vi "Read Serial Settings.vi"(8 "error in":errorcluster, 11 "4124 in":refnum<class "4124.lvclass">) -> (0 "error out":errorcluster, 2 "Serial Configuration":T1={"Baud Rate"=9600, "Parity"=0, "Data Bits"=7, "Stop Bits"=10, "Flow Control"=0} {"Flow Control" items=["None", "XON/XOFF", "RTS/CTS", "XON/XOFF & RTS/CTS", "DTR/DSR", "XON/XOFF & DTR/DSR"]; "Stop Bits" items=["1.0"=10, "1.5"=15, "2.0"=20]; "Data Bits" items=["7"=7, "8"=8]; "Parity" items=["None", "Odd", "Even", "Mark", "Space"]; "Baud Rate" items=["300"=300, "600"=600, "1200"=1200, "2400"=2400, "4800"=4800, "9600"=9600, "19200"=19200]}, 3 "4124 out":refnum<class "4124.lvclass">)   [LabVIEW 2018, in "4124.lvlib" / "4124.lvclass"]
uses:
  4124.lvclass
  builds/Power_Supply.lvlibp/Power Supply.lvclass
  builds/Configuration.lvlibp/Configuration.lvclass
  C:/Users/Ron.Dexter.LUMINARTECH/Desktop/builds/Power_Supply.lvlibp/Power Supply.lvclass
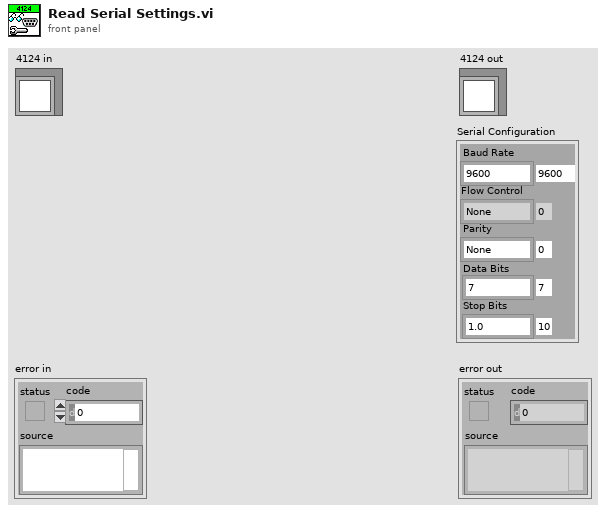
[diagram p1: front panel]
types:
  T1 = cluster{"Baud Rate":u32, "Parity":u16, "Data Bits":u16, "Stop Bits":u16, "Flow Control":u16}
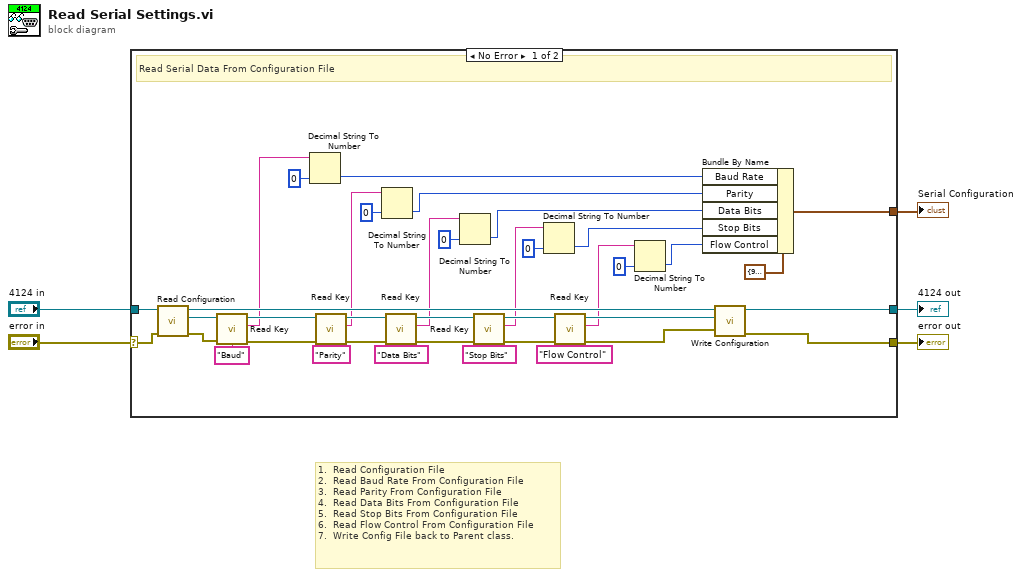
[diagram p0: block diagram]
diagram:
  # "1.  Read Configuration File\n2.  Read Baud Rate From Configuration File\n3.  Read Parity From Configuration File\n4.  Read Data Bits From Configuration File\n5.  Read Stop Bits From Configuration File\n6.  Read Flow Control From Configuration File\n7.  Write Config File back to Parent class."
  n1 = case shown="No Error" "error in" {
    selector: "error in" -> [w20 w46]
    tunnel: [w6 w46] -> w4
    tunnel: [w23 w45] -> w2
    tunnel: "4124 in" -> [w24 w45]
    tunnel: [w21 _] -> w1
    frame No Error {
      # "Read Serial Data From Configuration File"
      n2 = call "Read Configuration.vi"("error in (no error)"=w20, "Power Supply in"=w24) -> ("error out"=w43:errorcluster, "Configuration"=w44:refnum<class "Configuration.lvclass">, "Power Supply out"=w31:refnum<class "4124.lvclass">)  [unwired: 7 in]
      n3 = call "Read Key.vi"("Key:"="Baud", "error in"=w43, "Configuration in"=w44) -> ("error out"=w29:errorcluster, "Value"=w19:string, "Configuration out"=w35:refnum<class "Configuration.lvclass">)  [unwired: 6 in]
      n4 = Decimal String To Number(string=w19, default (0L)=u32 0 ("default (0 I32)")) -> (number=w18:u32)  [unwired: 1 in, 1 out]
      n5 = call "Read Key.vi"("Key:"="Parity", "error in"=w29, "Configuration in"=w35) -> ("error out"=w28:errorcluster, "Value"=w17:string, "Configuration out"=w34:refnum<class "Configuration.lvclass">)  [unwired: 6 in]
      n6 = Decimal String To Number(string=w17, default (0L)=u16 0 ("default (0 I32)")) -> (number=w15:u16)  [unwired: 1 in, 1 out]
      n7 = call "Read Key.vi"("Key:"="Data Bits", "error in"=w28, "Configuration in"=w34) -> ("error out"=w27:errorcluster, "Value"=w14:string, "Configuration out"=w33:refnum<class "Configuration.lvclass">)  [unwired: 6 in]
      n8 = Decimal String To Number(string=w14, default (0L)=u16 0 ("default (0 I32)")) -> (number=w13:u16)  [unwired: 1 in, 1 out]
      n9 = call "Read Key.vi"("Key:"="Stop Bits", "error in"=w27, "Configuration in"=w33) -> ("error out"=w26:errorcluster, "Value"=w11:string, "Configuration out"=w32:refnum<class "Configuration.lvclass">)  [unwired: 6 in]
      n10 = Decimal String To Number(string=w11, default (0L)=u16 0 ("default (0 I32)")) -> (number=w10:u16)  [unwired: 1 in, 1 out]
      n11 = call "Read Key.vi"("Key:"="Flow Control", "error in"=w26, "Configuration in"=w32) -> ("error out"=w25:errorcluster, "Value"=w7:string, "Configuration out"=w30:refnum<class "Configuration.lvclass">)  [unwired: 6 in]
      n12 = Decimal String To Number(string=w7, default (0L)=u16 0 ("default (0 I32)")) -> (number=w8:u16)  [unwired: 1 in, 1 out]
      n13 = Bundle By Name(cluster=T1 {"Baud Rate"=9600, "Parity"=0, "Data Bits"=7, "Stop Bits"=10, "Flow Control"=0} ("Serial Configuration"), "Baud Rate"=w18, "Parity"=w15, "Data Bits"=w13, "Stop Bits"=w10, "Flow Control"=w8) -> (w21:T1)
      n14 = call "Write Configuration.vi"("error in (no error)"=w25, "Configuration"=w30, "Power Supply in"=w31) -> ("error out"=w6:errorcluster, "Power Supply out"=w23:refnum<class "4124.lvclass">)  [unwired: 7 in]
    }
    frame Error {
      # "Return Error and Default Serial Configuration"
    }
  }
  "error out" <- w4
  "4124 out" <- w2
  "Serial Configuration" <- w1
